vi "move-and-measure_NI - stability.vi"(0 "fpga-ref-in":refnum<k20>, 1 "XY-in":dbl[](array[numeric]), 2 "bar-note":u8, 7 "stage-refs":T1, 11 "stage-error-in":errorcluster, 12 "counter-in":dbl format="%#_13g", 13 "meas#":dbl) -> (3 "measured-point out":dbl[](array[numeric]), 4 "logfile-line-out":string, 6 "iCorr-out":dbl, 14 "counter-out":dbl, 15 "stage-error-out":errorcluster)   [LabVIEW 2024]
uses:
  C:/Users/hpDIRC/Desktop/eic_dirc_daq-LabVIEW_new/Thorlabs.MotionControl.IntegratedStepperMotorsCLI.dll
  Thorlabs.MotionControl.IntegratedStepperMotorsCLI.dll
  C:/Users/hpDIRC/Desktop/eic_dirc_daq-LabVIEW_new/Thorlabs.MotionControl.Benchtop.StepperMotorCLI.dll
  Thorlabs.MotionControl.Benchtop.StepperMotorCLI.dll
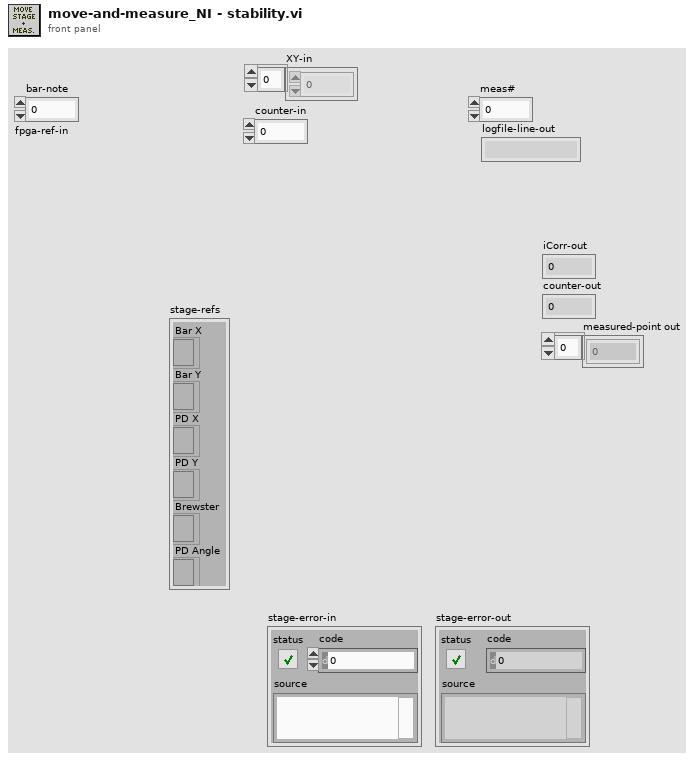
[diagram p1: front panel]
types:
  T1 = cluster{"Bar X":refnum<k24>, "Bar Y":refnum<k24>, "PD X":refnum<k24>, "PD Y":refnum<k24>, "Brewster":refnum<k24>, "PD Angle":refnum<k24>}
  T2 = cluster{"Bar X":dbl, "Bar Y":dbl, "PD X":dbl, "PD Y":dbl, "BMA":dbl, "PDA":dbl}
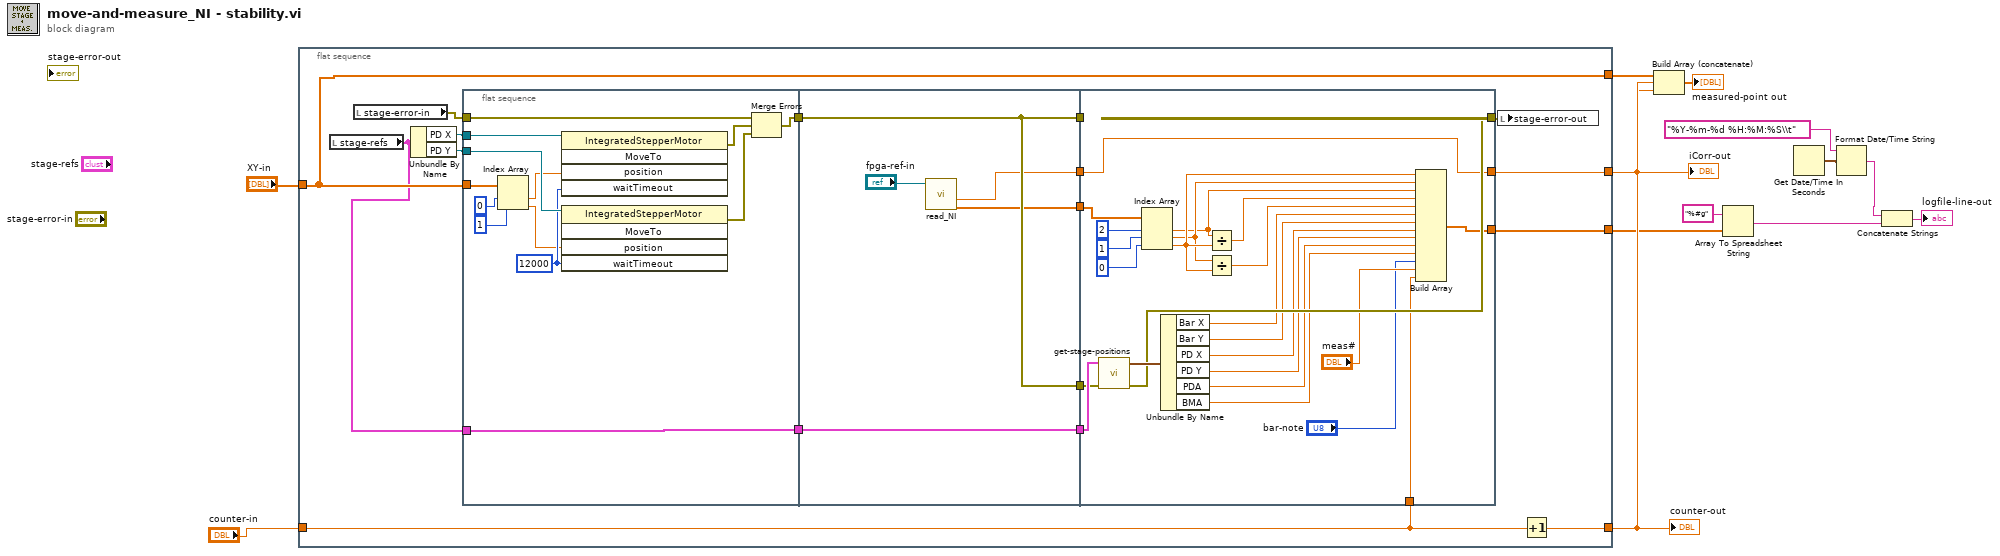
[diagram p0: block diagram]
diagram:
  n1 = flat-sequence {
    tunnel: [w28] -> w9
    tunnel: "XY-in" -> [w24]
    tunnel: "counter-in" -> [w15]
    tunnel: [w16] -> w8
    tunnel: [w24] -> w10
    tunnel: [w14] -> w5
    frame #0 {
      n2 = local read "stage-refs"() -> (w18:T1)
      n3 = local read "stage-error-in"() -> (w26:errorcluster)
      n4 = Unbundle By Name(w18) -> ("PD X"=w30:refnum<k24>, "PD Y"=w29:refnum<k24>)
      n5 = flat-sequence {
        tunnel: w30 -> [w41]
        tunnel: w29 -> [w40]
        tunnel: w26 -> [w34]
        tunnel: w24 -> [w32]
        tunnel: [w33] -> w25
        tunnel: [w31] -> w19
        tunnel: w18 -> [w31]
        tunnel: w25 -> [w47]
        tunnel: [w45] -> w23
        tunnel: [w47] -> w22
        tunnel: [w46] -> w21
        tunnel: [w48] -> w20
        tunnel: w19 -> [w48]
        tunnel: [w47] -> w17
        tunnel: [w63] -> w27
        tunnel: [w51] -> w28
        tunnel: w23 -> [w51]
        tunnel: w22 -> [_]
        tunnel: w21 -> [w69]
        tunnel: w20 -> [w65]
        tunnel: w17 -> [w64]
        tunnel: w15 -> [w56]
        tunnel: [w54] -> w14
        frame #0 {
          w39 = 12000 ("waitTimeout")
          n6 = Index Array(array=w32, index #1=0 ("index"), index #2=1 ("index")) -> (element #1=w36:dbl, element #2=w35:dbl)
          n7 = invoke class="IntegratedStepperMotor" method="MoveTo"(reference=w41, "position"=w36, "waitTimeout"=w39) -> (error out=w43:errorcluster)  [unwired: 2 in, 4 out]
          n8 = invoke class="IntegratedStepperMotor" method="MoveTo"(reference=w40, "position"=w35, "waitTimeout"=w39) -> (error out=w42:errorcluster)  [unwired: 2 in, 4 out]
          n9 = Merge Errors(w34, w43, w42) -> (w33:errorcluster)
        }
        frame #1 {
          n10 = call "read_NI.vi"("fpga-ref-in"="fpga-ref-in") -> ("all_pds"=w46:dbl[], "-pd3/pd1"=w45:dbl)  [unwired: 6 in, 3 out]
        }
        frame #2 {
          n11 = call "get-stage-positions.vi"("error in (no error)"=w64, "Cluster"=w65) -> ("error out"=w63:errorcluster, "stage positions"=w66:T2)  [unwired: 8 in]
          n12 = Index Array(array=w69, index #1=2 ("index"), index #2=1 ("index"), index #3=0 ("index")) -> (element #1=w50:dbl, element #2=w52:dbl, element #3=w53:dbl)
          n13 = Unbundle By Name(w66) -> ("Bar X"=w62:dbl, "Bar Y"=w61:dbl, "PD X"=w60:dbl, "PD Y"=w59:dbl, "PDA"=w58:dbl, "BMA"=w57:dbl)
          n14 = Divide(x=w50, y=w53) -> (x/y=w68:dbl)
          n15 = Divide(x=w52, y=w53) -> (x/y=w67:dbl)
          n16 = Build Array(w53, w52, w50, w68, w67, w62, w61, w60, w59, w58, w57, "bar-note", "meas#", w56) -> (w54:dbl[])
        }
      }
      n17 = local write "stage-error-out"(w27) -> ()
      n18 = Increment(x=w15) -> (x+1=w16:dbl)
    }
  }
  n19 = Build Array (concatenate)(w10, w9, w8) -> (→"measured-point out":dbl[])
  n20 = Array To Spreadsheet String(array=w5, 3:"%#g" ("format string")) -> (spreadsheet string=w3:string)  [unwired: 1 in]
  n21 = Get Date/Time In Seconds() -> (seconds since 1Jan1904=w7:timestamp)
  n22 = Format Date/Time String(time format string (%c)="%Y-%m-%d %H:%M:%S\\t", seconds (now)=w7) -> (date/time string=w2:string)  [unwired: 1 in]
  n23 = Concatenate Strings(w2, w3) -> (→"logfile-line-out":string)
  "iCorr-out" <- w9
  "counter-out" <- w8
